vi "Pcre2ErrorNull.vi"(7 "IsPointer? (F)":bool, 9 "error in":errorcluster, 10 "What":string) -> (1 "error out":errorcluster)   [LabVIEW 2021, in "libpcre2-8.lvlib"]
uses:
  libpcre2-8.lvlib
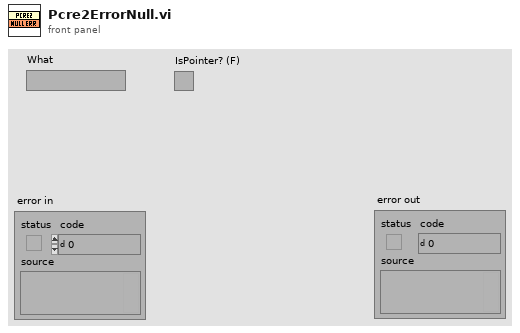
[diagram p1: front panel]
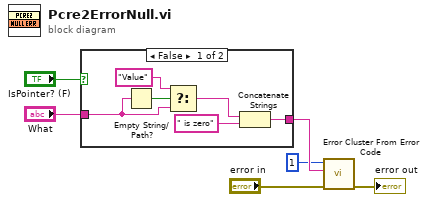
[diagram p0: block diagram]
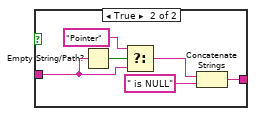
[diagram p2: hidden frame]
diagram:
  n1 = case shown="False" "IsPointer? (F)" {
    tunnel: [w7 w18] -> w4
    tunnel: "What" -> [w8 w16]
    frame False {
      n2 = Empty String/Path?(string/path=w8) -> (empty?=w12:bool)
      n3 = Select(t="Value", s=w12, f=w8) -> (s? t:f=w11:string)
      n4 = Concatenate Strings(w11, " is zero" ("string")) -> (w7:string)
    }
    frame True {
      n5 = Empty String/Path?(string/path=w16) -> (empty?=w17:bool)
      n6 = Select(t="Pointer", s=w17, f=w16) -> (s? t:f=w15:string)
      n7 = Concatenate Strings(w15, " is NULL" ("string")) -> (w18:string)
    }
  }
  n8 = call <vilib>:"Error Cluster From Error Code.vi"("error in (no error)"="error in", "error message (\"\")"=w4, "error code (0)"=1 ("code (0)")) -> ("error out"=→"error out":errorcluster)  [unwired: 6 in]
